vi "getZThXThYBTor.vi"(10 "PosMeas_ZeroOffset":fxp<+/-,25,5>[](array[numeric])=[0.0, 0.0, 0.0, 0.0, 0.0], 11 "PosMeas_Array In":fxp<+/-,25,5>[](array[numeric])=[0.0, 0.0, 0.0, 0.0, 0.0, 0.0, 0.0, 0.0, 0.0, 0.0, 0.0, 0.0, 0.0]) -> (3 "Z,ThX,ThY,B,Tor_out":fxp<+/-,25,5>[](array[numeric]))   [LabVIEW 2020, in "PositionMeas.lvlib"]
doc: "Returns the Z, ThX, ThY, Bow, and Torsion mode measurements based on position sensor data"
uses:
  PositionMeas.lvlib
  <vilib>/Platform/TimedLoop/XDataNode/XDataNode.xnode
  <vilib>/Platform/TimedLoop/XDataNode/nitl_modes.ctl
  <vilib>/Platform/TimedLoop/XDataNode/XDNodeRunTimeDep.lvlib
  <vilib>/Platform/TimedLoop/XDataNode/wakeup.ctl
  <vilib>/Platform/TimedLoop/XDataNode/timing_clust.ctl
  <vilib>/rvi/FXPMathLib/FxpSub/XNode/nifxpmath_Sub.xnode
  <vilib>/rvi/FXPMathLib/sim/FxpSim.dll
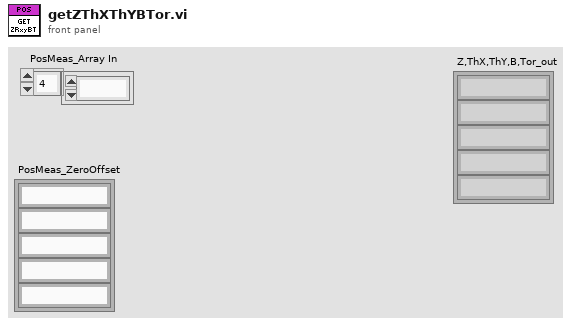
[diagram p1: front panel]
types:
  T1 = typedef "XDNodeRunTimeDep.lvlib/timing_clust.ctl" = cluster{"Expected End [f-1]":u64, "Actual End [f-1]":u64, "Finished Late? [f-1]":bool, "Expected End [i-1]":u64, "Actual End [i-1]":u64, "Finished Late? [i-1]":bool, "Expected Start [i]":u64, "Actual Start [i]":u64, "Expected Start [f]":u64, "Actual Start [f]":u64, "Source Name":string, "Structure Name":string, "Period":i64, "Deadline":i64, "Offset":i64, "Start":i64, "Priority":i32, "Timeout":i32, "Mode":T2, "Wakeup Reason":T3, "Error":errorcluster, "Source Type":string, "Secondary Source Type":string, "Global End Time":u64, "Global Start Time":u64, "Frame Duration":u64, "Iteration Duration":u64, "Assigned CPU":i32, "I/O Scan Engine Mode":u32}
  T2 = typedef "XDNodeRunTimeDep.lvlib/nitl_modes.ctl" = enum32{"No Change", "Process missed periods, maintain original phase", "Discard missed periods, maintain original phase", "Process missed periods, ignore original phase", "Discard missed periods, ignore original phase"}
  T3 = typedef "XDNodeRunTimeDep.lvlib/wakeup.ctl" = enum32{"Normal", "Aborted", "Asynchronous wakeup", "Timing source error", "Timed loop error", "Timeout"}
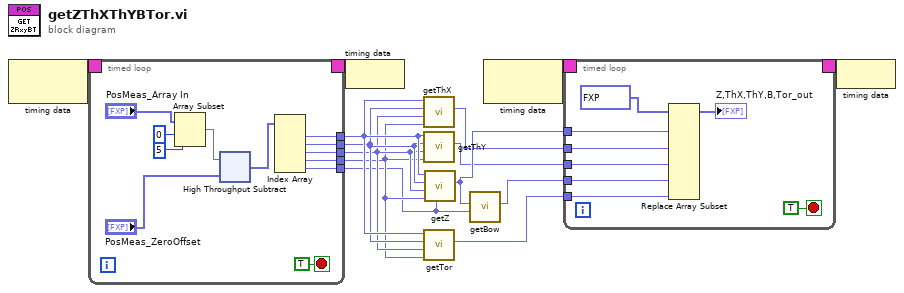
[diagram p0: block diagram]
diagram:
  n1 = node-c288() -> (w8:T1)  [unwired: 1 in]
  n2 = timed-loop {
    timing: w8 -> [_]
    timing-out: [_] -> w7
    tunnel: [w26] -> w6
    tunnel: [w25] -> w5
    tunnel: [w24] -> w4
    tunnel: [w23] -> w3
    tunnel: [w22] -> w1
    stop <- TRUE stop-if-true
    n3 = Array Subset(array="PosMeas_Array In", index=0, length=5) -> (w17:fxp<+/-,25,5>[])
    n4 = xnode ("High Throughput Subtract")("x"=w17, "y"="PosMeas_ZeroOffset") -> ("x-y"=w15:fxp<+/-,25,5>[])
    n5 = Index Array(array=w15) -> (element #1=w26:fxp<+/-,25,5>, element #2=w25:fxp<+/-,25,5>, element #3=w24:fxp<+/-,25,5>, element #4=w23:fxp<+/-,25,5>, element #5=w22:fxp<+/-,25,5>)  [unwired: 5 in]
  }
  n6 = node-c288(w7) -> ()
  n7 = call "getThX.vi"("SW"=w3, "NW"=w4, "NE"=w5, "SE"=w6) -> ("ThX"=w11:fxp<+/-,25,5>)  [unwired: 7 in]
  n8 = call "getThY.vi"("SW"=w3, "NW"=w4, "NE"=w5, "SE"=w6) -> ("ThY"=w10:fxp<+/-,25,5>)  [unwired: 7 in]
  n9 = call "getTor.vi"("SW"=w3, "NW"=w4, "NE"=w5, "SE"=w6) -> ("Bow_diag"=w2:fxp<+/-,25,5>)  [unwired: 7 in]
  n10 = call "getZ.vi"("CI"=w1, "SW"=w3, "NW"=w4, "NE"=w5, "SE"=w6) -> ("Z"=w12:fxp<+/-,25,5>)  [unwired: 6 in]
  n11 = call "getBow.vi"("CI"=w1, "Z"=w12) -> ("Bow"=w9:fxp<+/-,25,5>)  [unwired: 9 in]
  n12 = node-c288() -> (w14:T1)  [unwired: 1 in]
  n13 = timed-loop {
    timing: w14 -> [_]
    timing-out: [_] -> w13
    tunnel: w12 -> [w36]
    tunnel: w11 -> [w35]
    tunnel: w10 -> [w34]
    tunnel: w9 -> [w33]
    tunnel: w2 -> [w29]
    stop <- TRUE stop-if-true
    n14 = Replace Array Subset(array=fxp<+/-,25,5>[] [0.0, 0.0, 0.0, 0.0, 0.0], new element #1=w36, new element #2=w35, new element #3=w34, new element #4=w33, new element #5=w29) -> (→"Z,ThX,ThY,B,Tor_out":fxp<+/-,25,5>[])  [unwired: 5 in]
  }
  n15 = node-c288(w13) -> ()
